vi "Move new unbundler WRT Terminal.vi"(6 "Offset":i32=-15, 8 "error in":errorcluster, 9 "New objects created":refnum<vi>[](array[refnum]), 10 "Named Un/Bundler Ref":refnum<vi>, 11 "Terminal Data Cluster":T1) -> (0 "error out":errorcluster)   [LabVIEW 2023]
doc: "Because a bundler will expand to the right once its labels are set, and we want to place the bundler to the left of a sink terminal, this VI will adjust the new objects created (a bundler and optional constant) to be positioned the correct offset from the affected terminal. Offset is by default -15px.\n\nThis is not needed for bundlers on source terminals, so we ignore those."
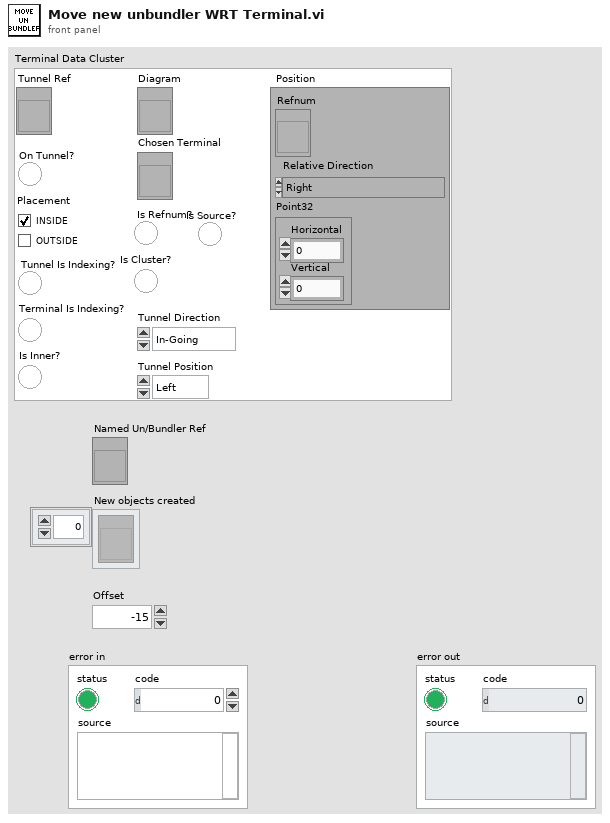
[diagram p1: front panel]
types:
  T1 = cluster{"Tunnel Ref":refnum<vi>, "On Tunnel?":bool, "Placement":enum32{"Choice 1", "Choice 2"}, "Tunnel Is Indexing?":bool, "Diagram":refnum<vi>, "Position":cluster{"Refnum":refnum<vi>, "Relative Direction":enum32{"Right", "Left", "Top", "Bottom", "Top Right", "Top Left", "Bottom Right", "Bottom Left"}, "Point32":cluster{"Horizontal":i32, "Vertical":i32}}, "Chosen Terminal":refnum<vi>, "Is Refnum?":bool, "Is Cluster?":bool, "Is Source?":bool, "Tunnel Direction":enum16{"In-Going", "Out-Going"}, "Tunnel Position":enum16{"Left", "Top", "Right", "Bottom"}, "Is Inner?":bool, "Terminal Is Indexing?":bool}
  T2 = typedef "LVPositionTypeDef.ctl" = cluster{"Left":i32, "Top":i32}
  T3 = typedef "LVRectTypeDef.ctl" = cluster{"Left":i16, "Top":i16, "Right":i16, "Bottom":i16}
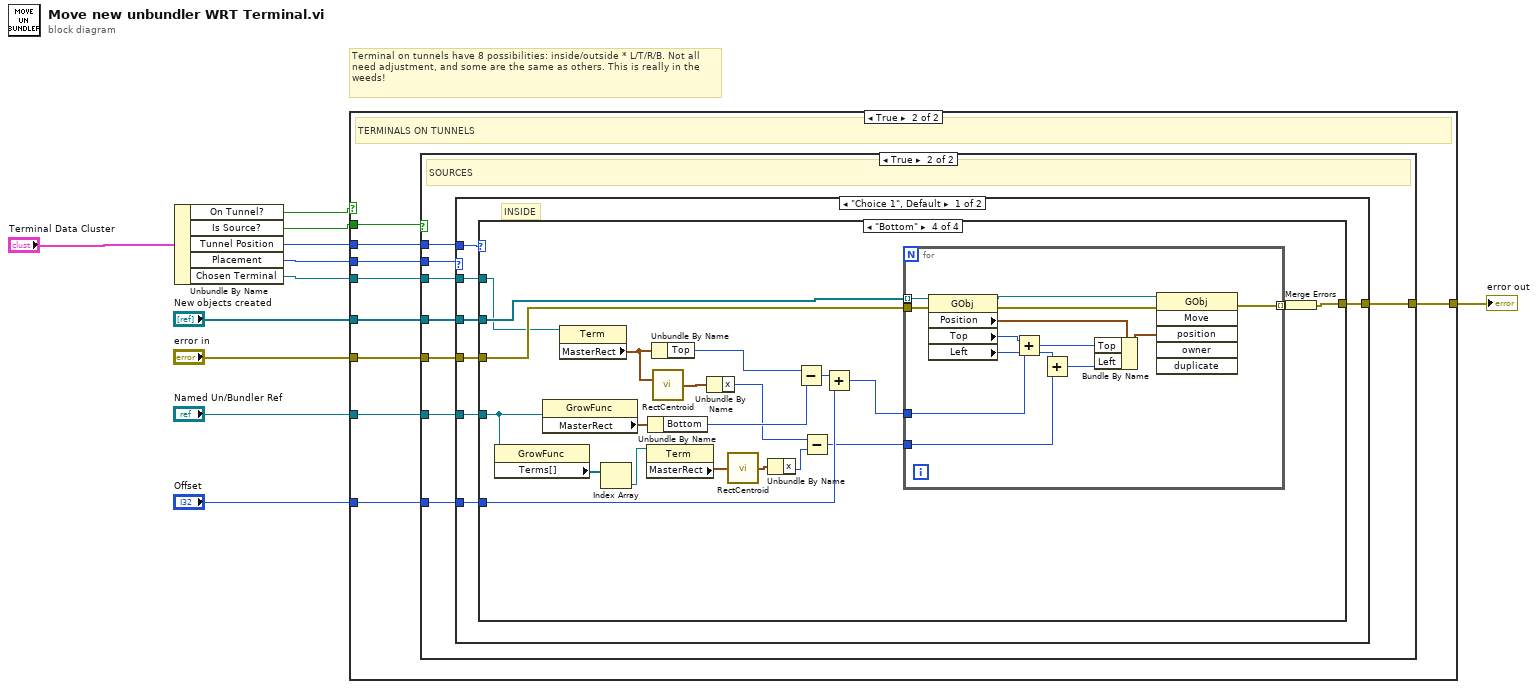
[diagram p0: block diagram]
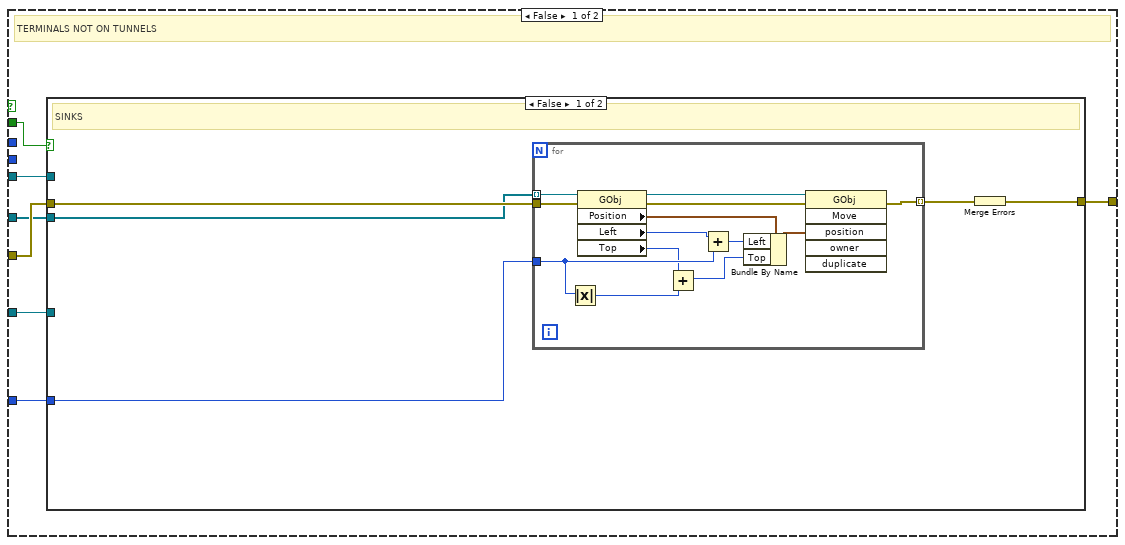
[diagram p2: hidden frame]
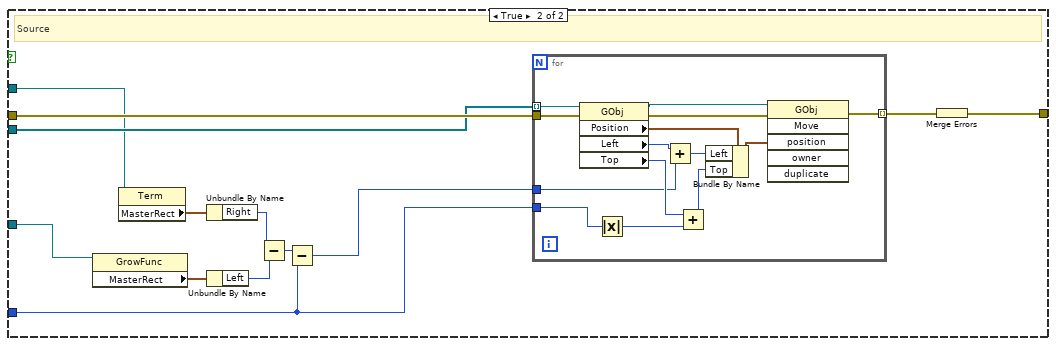
[diagram p3: hidden frame]
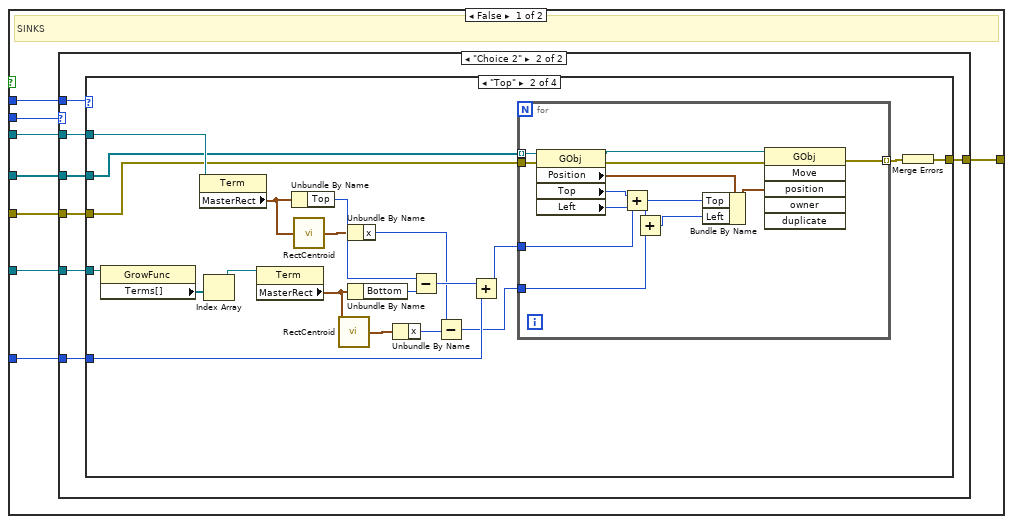
[diagram p4: hidden frame]
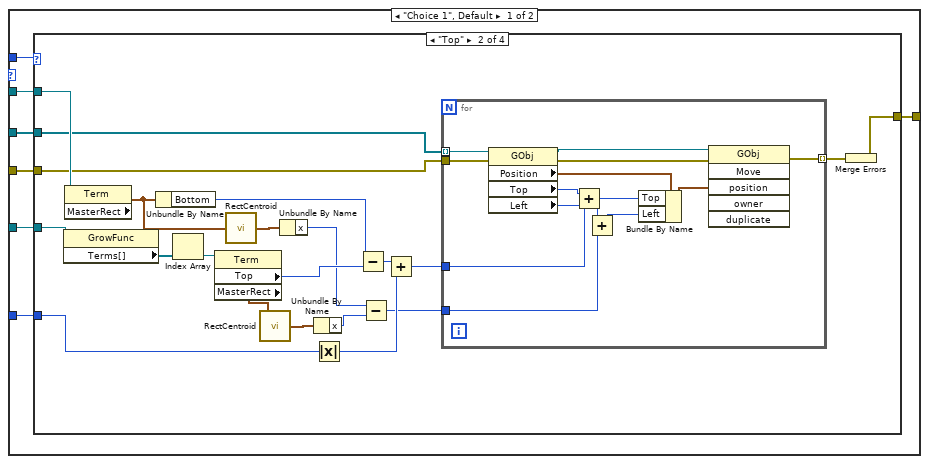
[diagram p5: hidden frame]
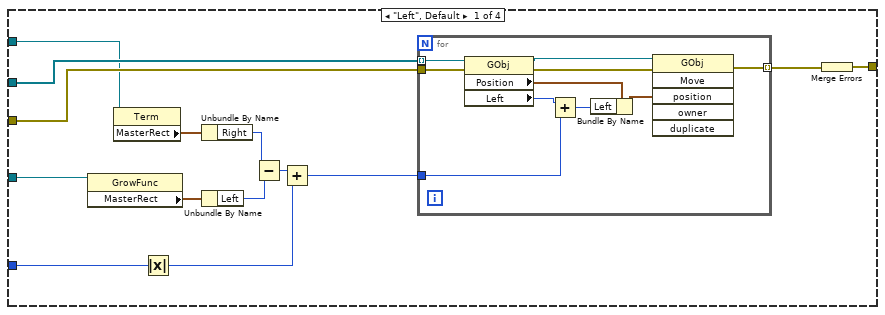
[diagram p6: hidden frame]
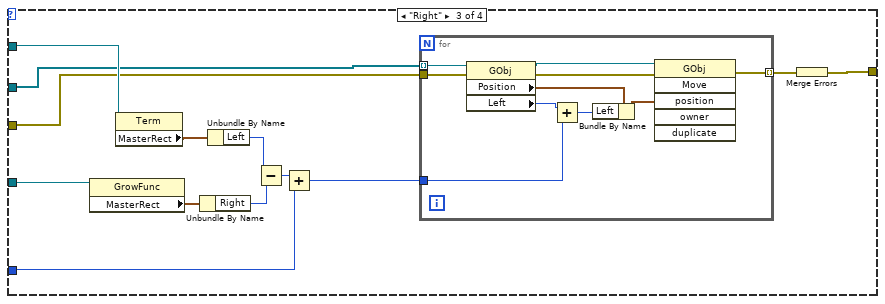
[diagram p7: hidden frame]
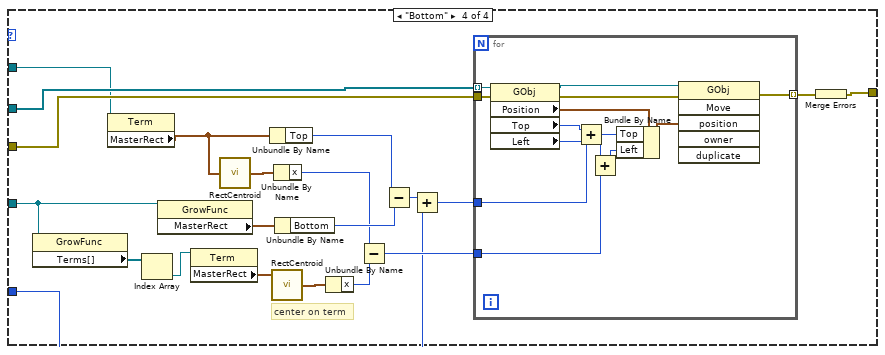
[diagram p8: hidden frame]
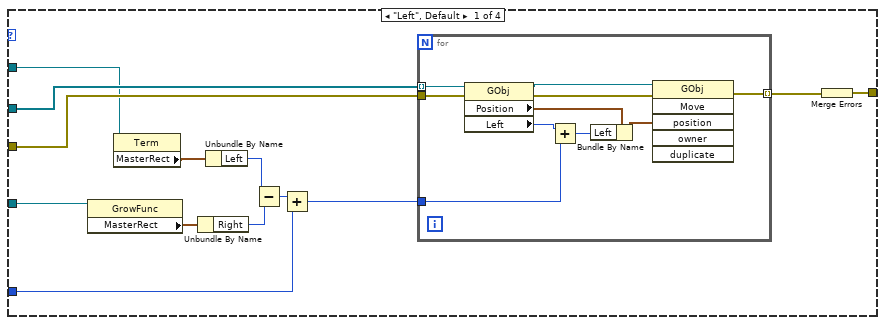
[diagram p9: hidden frame]
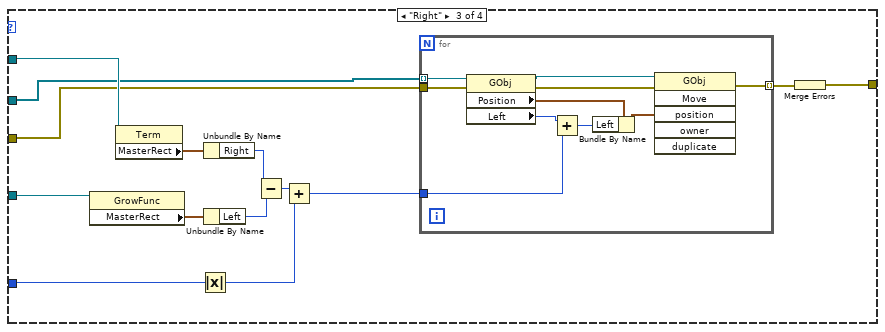
[diagram p10: hidden frame]
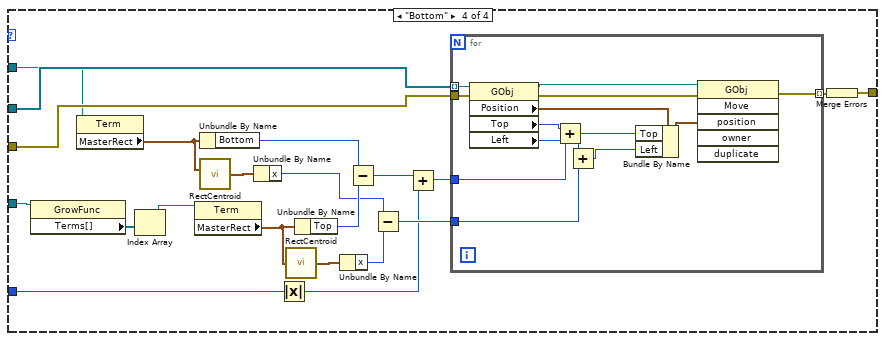
[diagram p11: hidden frame]
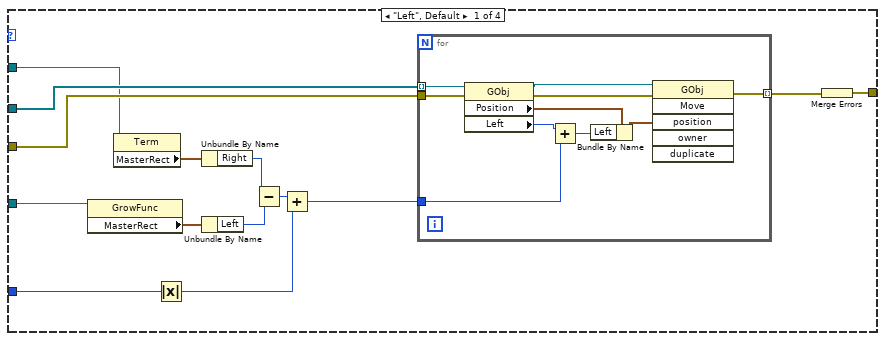
[diagram p12: hidden frame]
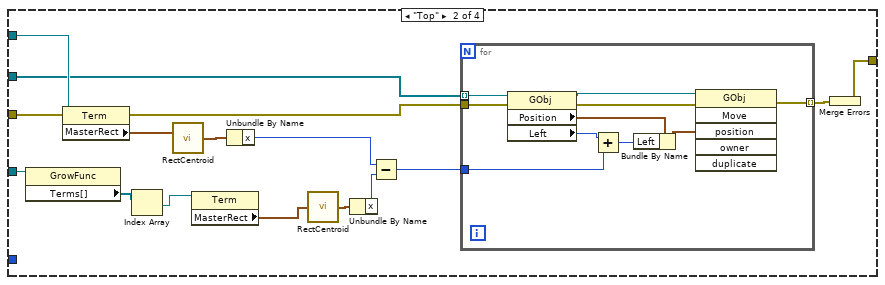
[diagram p13: hidden frame]
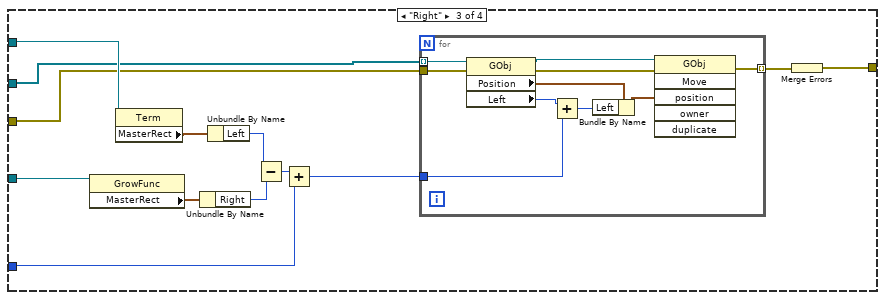
[diagram p14: hidden frame]
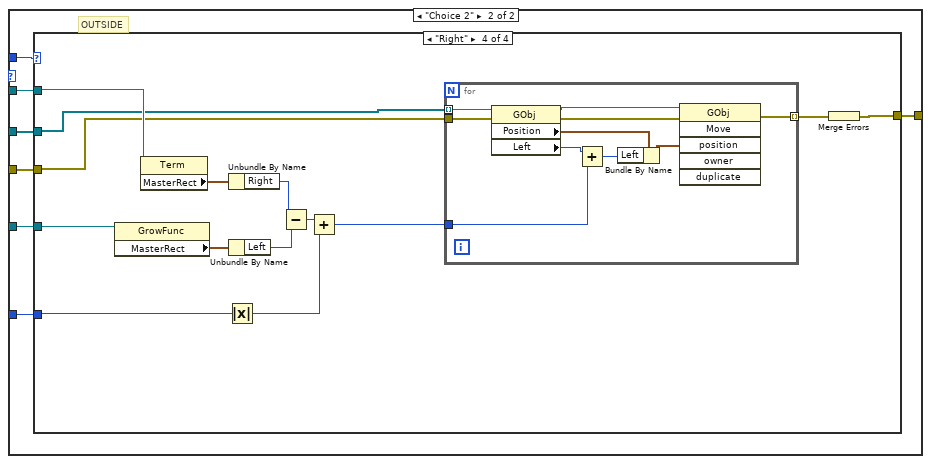
[diagram p15: hidden frame]
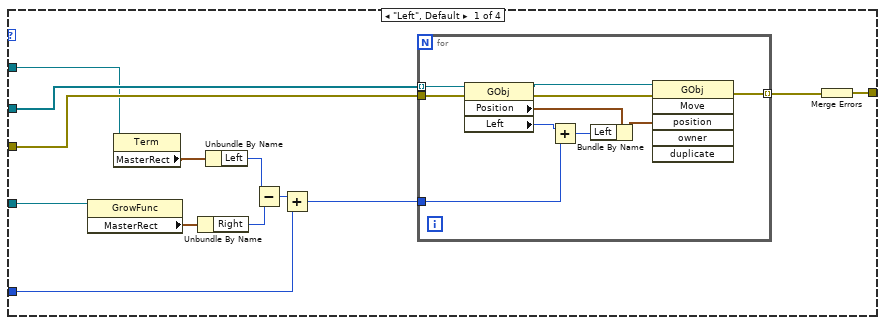
[diagram p16: hidden frame]
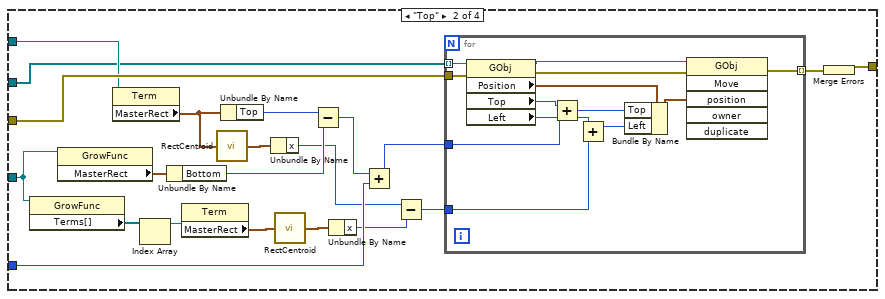
[diagram p17: hidden frame]
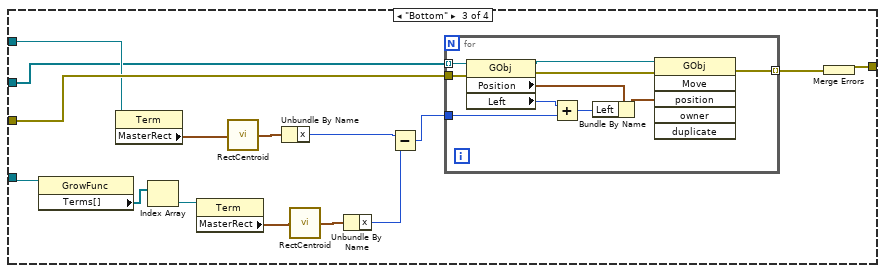
[diagram p18: hidden frame]
diagram:
  # "Terminal on tunnels have 8 possibilities: inside/outside * L/T/R/B. Not all need adjustment, and some are the same as others. This is really in the weeds!"
  n1 = Unbundle By Name("Terminal Data Cluster") -> ("On Tunnel?"=w5:bool, "Is Source?"=w4:bool, "Tunnel Position"=w3:enum16{"Left", "Top", "Right", "Bottom"}, "Placement"=w2:enum32{"Choice 1", "Choice 2"}, "Chosen Terminal"=w6:refnum<vi>)
  n2 = case shown="True" w5 {
    tunnel: "Offset" -> [w18 w64]
    tunnel: "Named Un/Bundler Ref" -> [w17 w66]
    tunnel: [w16 w69] -> w9
    tunnel: "error in" -> [w15 w68]
    tunnel: w4 -> [w14 w72]
    tunnel: w6 -> [w13 w65]
    tunnel: w3 -> [_ w71]
    tunnel: w2 -> [_ w70]
    tunnel: "New objects created" -> [w12 w67]
    frame False {
      # "TERMINALS NOT ON TUNNELS"
      n3 = case shown="False" w14 {
        tunnel: w18 -> [w23 w38]
        tunnel: w17 -> [_ w39]
        tunnel: w13 -> [_ w40]
        tunnel: [w21 w48] -> w16
        tunnel: w15 -> [w20 w47]
        tunnel: w12 -> [w19 w46]
        frame False {
          # "SINKS"
          n4 = for {
            tunnel: w19 -> [w36] mode=indexing
            tunnel: w23 -> [w27]
            tunnel: w20 -> [w30]
            tunnel: [w28] -> w22 mode=indexing
            n5 = Absolute Value(x=w27) -> (abs(x)=w24:i32)
            n6 = property class="GObj"(reference=w36, error in=w30) -> (reference out=w35:refnum<vi>, error out=w29:errorcluster, "Position"=w33:T2, "Left"=w34:i32, "Top"=w26:i32)
            n7 = Add(x=w26, y=w24) -> (x+y=w25:i32)
            n8 = Add(x=w34, y=w27) -> (x+y=w32:i32)
            n9 = Bundle By Name(cluster=w33, "Left"=w32, "Top"=w25) -> (w31:T2)
            n10 = invoke class="GObj" method="Move"(reference=w35, error in=w29, "position"=w31) -> (error out=w28:errorcluster)  [unwired: 3 in, 5 out]
          }
          n11 = Merge Errors(w22) -> (w21:errorcluster)
        }
        frame True {
          # "Source"
          n12 = property class="GrowFunc"(reference=w39) -> ("MasterRect"=w44:T3)  [unwired: 1 in, 2 out]
          n13 = property class="Term"(reference=w40) -> ("MasterRect"=w43:T3)  [unwired: 1 in, 2 out]
          n14 = Unbundle By Name(w43) -> ("Right"=w42:i16)
          n15 = Unbundle By Name(w44) -> ("Left"=w41:i16)
          n16 = Subtract(x=w42, y=w41) -> (x-y=w45:i16)
          n17 = Subtract(x=w45, y=w38) -> (x-y=w37:i32)
          n18 = for {
            tunnel: w46 -> [w63] mode=indexing
            tunnel: w38 -> [w50]
            tunnel: w47 -> [w57]
            tunnel: [w55] -> w49 mode=indexing
            tunnel: w37 -> [w51]
            n19 = property class="GObj"(reference=w63, error in=w57) -> (reference out=w62:refnum<vi>, error out=w56:errorcluster, "Position"=w60:T2, "Left"=w61:i32, "Top"=w53:i32)
            n20 = Absolute Value(x=w50) -> (abs(x)=w54:i32)
            n21 = Add(x=w61, y=w51) -> (x+y=w59:i32)
            n22 = Add(x=w53, y=w54) -> (x+y=w52:i32)
            n23 = Bundle By Name(cluster=w60, "Left"=w59, "Top"=w52) -> (w58:T2)
            n24 = invoke class="GObj" method="Move"(reference=w62, error in=w56, "position"=w58) -> (error out=w55:errorcluster)  [unwired: 3 in, 5 out]
          }
          n25 = Merge Errors(w49) -> (w48:errorcluster)
        }
      }
    }
    frame True {
      # "TERMINALS ON TUNNELS"
      n26 = case shown="True" w72 {
        tunnel: w71 -> [w80 w331]
        tunnel: w70 -> [w79 w330]
        tunnel: [w78 w324] -> w69
        tunnel: w68 -> [w77 w327]
        tunnel: w67 -> [w76 w328]
        tunnel: w66 -> [w75 w326]
        tunnel: w65 -> [w74 w329]
        tunnel: w64 -> [w73 w325]
        frame False {
          # "SINKS"
          n27 = case shown="\"Choice 2\"" w79 {
            tunnel: w80 -> [w87 w209]
            tunnel: [w81 w208] -> w78
            tunnel: w77 -> [w84 w207]
            tunnel: w76 -> [w85 w206]
            tunnel: w75 -> [w82 w205]
            tunnel: w74 -> [w86 w204]
            tunnel: w73 -> [w83 w203]
            frame "Choice 1", Default {
              n28 = case shown="\"Top\"" w87 {
                tunnel: [w96 w126 w158 w180] -> w81
                tunnel: w84 -> [w100 w128 w155 w182]
                tunnel: w85 -> [w101 w127 w156 w183]
                tunnel: w82 -> [w99 w125 w154 w179]
                tunnel: w86 -> [w98 w129 w157 w181]
                tunnel: w83 -> [w97 w120 w153 w173]
                frame "Left", Default {
                  n29 = property class="GrowFunc"(reference=w99) -> ("MasterRect"=w94:T3)  [unwired: 1 in, 2 out]
                  n30 = property class="Term"(reference=w98) -> ("MasterRect"=w93:T3)  [unwired: 1 in, 2 out]
                  n31 = Absolute Value(x=w97) -> (abs(x)=w88:i32)
                  n32 = Unbundle By Name(w93) -> ("Right"=w92:i16)
                  n33 = Unbundle By Name(w94) -> ("Left"=w91:i16)
                  n34 = Subtract(x=w92, y=w91) -> (x-y=w95:i16)
                  n35 = Add(x=w95, y=w88) -> (x+y=w90:i32)
                  n36 = for {
                    tunnel: w90 -> [w109]
                    tunnel: [w104] -> w89 mode=indexing
                    tunnel: w101 -> [w103] mode=indexing
                    tunnel: w100 -> [w102]
                    n37 = property class="GObj"(reference=w103, error in=w102) -> (reference out=w111:refnum<vi>, error out=w105:errorcluster, "Position"=w108:T2, "Left"=w110:i32)
                    n38 = Add(x=w110, y=w109) -> (x+y=w107:i32)
                    n39 = Bundle By Name(cluster=w108, "Left"=w107) -> (w106:T2)
                    n40 = invoke class="GObj" method="Move"(reference=w111, error in=w105, "position"=w106) -> (error out=w104:errorcluster)  [unwired: 3 in, 5 out]
                  }
                  n41 = Merge Errors(w89) -> (w96:errorcluster)
                }
                frame "Top" {
                  n42 = property class="GrowFunc"(reference=w125) -> ("Terms[]"=w124:refnum<vi>[])  [unwired: 1 in, 2 out]
                  n43 = property class="Term"(reference=w129) -> ("MasterRect"=w114:T3)  [unwired: 1 in, 2 out]
                  n44 = Unbundle By Name(w114) -> ("Bottom"=w118:i16)
                  n45 = Index Array(array=w124) -> (element=w123:refnum<vi>)  [unwired: 1 in]
                  n46 = property class="Term"(reference=w123) -> ("Top"=w122:i32, "MasterRect"=w115:T3)  [unwired: 1 in, 2 out]
                  n47 = call <vilib>:"RectCentroid.vi"("rect"=w114) -> ("point"=w117:cluster{"x":i16, "y":i16})
                  n48 = call <vilib>:"RectCentroid.vi"("rect"=w115) -> ("point"=w116:cluster{"x":i16, "y":i16})
                  n49 = Unbundle By Name(w117) -> ("x"=w113:i16)
                  n50 = Unbundle By Name(w116) -> ("x"=w112:i16)
                  n51 = Absolute Value(x=w120) -> (abs(x)=w121:i32)
                  n52 = Subtract(x=w118, y=w122) -> (x-y=w132:i32)
                  n53 = Subtract(x=w113, y=w112) -> (x-y=w119:i16)
                  n54 = Add(x=w132, y=w121) -> (x+y=w131:i32)
                  n55 = for {
                    tunnel: w131 -> [w143]
                    tunnel: [w138] -> w130 mode=indexing
                    tunnel: w128 -> [w137]
                    tunnel: w127 -> [w136] mode=indexing
                    tunnel: w119 -> [w134]
                    n56 = property class="GObj"(reference=w136, error in=w137) -> (reference out=w145:refnum<vi>, error out=w139:errorcluster, "Position"=w142:T2, "Top"=w144:i32, "Left"=w135:i32)
                    n57 = Add(x=w144, y=w143) -> (x+y=w141:i32)
                    n58 = Add(x=w135, y=w134) -> (x+y=w133:i32)
                    n59 = Bundle By Name(cluster=w142, "Top"=w141, "Left"=w133) -> (w140:T2)
                    n60 = invoke class="GObj" method="Move"(reference=w145, error in=w139, "position"=w140) -> (error out=w138:errorcluster)  [unwired: 3 in, 5 out]
                  }
                  n61 = Merge Errors(w130) -> (w126:errorcluster)
                }
                frame "Right" {
                  n62 = property class="GrowFunc"(reference=w154) -> ("MasterRect"=w151:T3)  [unwired: 1 in, 2 out]
                  n63 = property class="Term"(reference=w157) -> ("MasterRect"=w150:T3)  [unwired: 1 in, 2 out]
                  n64 = Unbundle By Name(w151) -> ("Right"=w148:i16)
                  n65 = Unbundle By Name(w150) -> ("Left"=w149:i16)
                  n66 = Subtract(x=w149, y=w148) -> (x-y=w152:i16)
                  n67 = Add(x=w152, y=w153) -> (x+y=w147:i32)
                  n68 = for {
                    tunnel: w156 -> [w168] mode=indexing
                    tunnel: w147 -> [w165]
                    tunnel: w155 -> [w161]
                    tunnel: [w159] -> w146 mode=indexing
                    n69 = property class="GObj"(reference=w168, error in=w161) -> (reference out=w167:refnum<vi>, error out=w160:errorcluster, "Position"=w164:T2, "Left"=w166:i32)
                    n70 = Add(x=w166, y=w165) -> (x+y=w163:i32)
                    n71 = Bundle By Name(cluster=w164, "Left"=w163) -> (w162:T2)
                    n72 = invoke class="GObj" method="Move"(reference=w167, error in=w160, "position"=w162) -> (error out=w159:errorcluster)  [unwired: 3 in, 5 out]
                  }
                  n73 = Merge Errors(w146) -> (w158:errorcluster)
                }
                frame "Bottom" {
                  # "center on term"
                  n74 = property class="GrowFunc"(reference=w179) -> ("Terms[]"=w178:refnum<vi>[])  [unwired: 1 in, 2 out]
                  n75 = property class="Term"(reference=w181) -> ("MasterRect"=w174:T3)  [unwired: 1 in, 2 out]
                  n76 = Index Array(array=w178) -> (element=w177:refnum<vi>)  [unwired: 1 in]
                  n77 = property class="GrowFunc"(reference=w179) -> ("MasterRect"=w188:T3)  [unwired: 1 in, 2 out]
                  n78 = property class="Term"(reference=w177) -> ("MasterRect"=w172:T3)  [unwired: 1 in, 2 out]
                  n79 = call <vilib>:"RectCentroid.vi"("rect"=w174) -> ("point"=w175:cluster{"x":i16, "y":i16})
                  n80 = Unbundle By Name(w174) -> ("Top"=w187:i16)
                  n81 = call <vilib>:"RectCentroid.vi"("rect"=w172) -> ("point"=w171:cluster{"x":i16, "y":i16})
                  n82 = Unbundle By Name(w175) -> ("x"=w170:i16)
                  n83 = Unbundle By Name(w188) -> ("Bottom"=w186:i16)
                  n84 = Unbundle By Name(w171) -> ("x"=w169:i16)
                  n85 = Subtract(x=w170, y=w169) -> (x-y=w176:i16)
                  n86 = Subtract(x=w187, y=w186) -> (x-y=w189:i16)
                  n87 = Add(x=w189, y=w173) -> (x+y=w185:i32)
                  n88 = for {
                    tunnel: w183 -> [w202] mode=indexing
                    tunnel: w185 -> [w199]
                    tunnel: w182 -> [w195]
                    tunnel: [w193] -> w184 mode=indexing
                    tunnel: w176 -> [w191]
                    n89 = property class="GObj"(reference=w202, error in=w195) -> (reference out=w201:refnum<vi>, error out=w194:errorcluster, "Position"=w198:T2, "Top"=w200:i32, "Left"=w192:i32)
                    n90 = Add(x=w200, y=w199) -> (x+y=w197:i32)
                    n91 = Add(x=w192, y=w191) -> (x+y=w190:i32)
                    n92 = Bundle By Name(cluster=w198, "Top"=w197, "Left"=w190) -> (w196:T2)
                    n93 = invoke class="GObj" method="Move"(reference=w201, error in=w194, "position"=w196) -> (error out=w193:errorcluster)  [unwired: 3 in, 5 out]
                  }
                  n94 = Merge Errors(w184) -> (w180:errorcluster)
                }
              }
            }
            frame "Choice 2" {
              n95 = case shown="\"Top\"" w209 {
                tunnel: [w210 w244 w279 w304] -> w208
                tunnel: w207 -> [w214 w246 w276 w303]
                tunnel: w206 -> [w215 w245 w277 w302]
                tunnel: w205 -> [w213 w242 w275 w300]
                tunnel: w204 -> [w212 w247 w278 w301]
                tunnel: w203 -> [w211 w243 w274 w299]
                frame "Left", Default {
                  n96 = property class="GrowFunc"(reference=w213) -> ("MasterRect"=w221:T3)  [unwired: 1 in, 2 out]
                  n97 = property class="Term"(reference=w212) -> ("MasterRect"=w220:T3)  [unwired: 1 in, 2 out]
                  n98 = Unbundle By Name(w221) -> ("Right"=w218:i16)
                  n99 = Unbundle By Name(w220) -> ("Left"=w219:i16)
                  n100 = Subtract(x=w219, y=w218) -> (x-y=w222:i16)
                  n101 = Add(x=w222, y=w211) -> (x+y=w217:i32)
                  n102 = for {
                    tunnel: w217 -> [w230]
                    tunnel: [w225] -> w216 mode=indexing
                    tunnel: w215 -> [w224] mode=indexing
                    tunnel: w214 -> [w223]
                    n103 = property class="GObj"(reference=w224, error in=w223) -> (reference out=w232:refnum<vi>, error out=w226:errorcluster, "Position"=w229:T2, "Left"=w231:i32)
                    n104 = Add(x=w231, y=w230) -> (x+y=w228:i32)
                    n105 = Bundle By Name(cluster=w229, "Left"=w228) -> (w227:T2)
                    n106 = invoke class="GObj" method="Move"(reference=w232, error in=w226, "position"=w227) -> (error out=w225:errorcluster)  [unwired: 3 in, 5 out]
                  }
                  n107 = Merge Errors(w216) -> (w210:errorcluster)
                }
                frame "Top" {
                  n108 = property class="GrowFunc"(reference=w242) -> ("Terms[]"=w234:refnum<vi>[])  [unwired: 1 in, 2 out]
                  n109 = property class="Term"(reference=w247) -> ("MasterRect"=w239:T3)  [unwired: 1 in, 2 out]
                  n110 = Index Array(array=w234) -> (element=w233:refnum<vi>)  [unwired: 1 in]
                  n111 = property class="Term"(reference=w233) -> ("MasterRect"=w236:T3)  [unwired: 1 in, 2 out]
                  n112 = Unbundle By Name(w239) -> ("Top"=w251:i16)
                  n113 = call <vilib>:"RectCentroid.vi"("rect"=w239) -> ("point"=w240:cluster{"x":i16, "y":i16})
                  n114 = call <vilib>:"RectCentroid.vi"("rect"=w236) -> ("point"=w237:cluster{"x":i16, "y":i16})
                  n115 = Unbundle By Name(w240) -> ("x"=w238:i16)
                  n116 = Unbundle By Name(w236) -> ("Bottom"=w250:i16)
                  n117 = Unbundle By Name(w237) -> ("x"=w235:i16)
                  n118 = Subtract(x=w251, y=w250) -> (x-y=w252:i16)
                  n119 = Subtract(x=w238, y=w235) -> (x-y=w241:i16)
                  n120 = Add(x=w252, y=w243) -> (x+y=w249:i32)
                  n121 = for {
                    tunnel: w249 -> [w263]
                    tunnel: [w258] -> w248 mode=indexing
                    tunnel: w246 -> [w257]
                    tunnel: w245 -> [w256] mode=indexing
                    tunnel: w241 -> [w254]
                    n122 = property class="GObj"(reference=w256, error in=w257) -> (reference out=w265:refnum<vi>, error out=w259:errorcluster, "Position"=w262:T2, "Top"=w264:i32, "Left"=w255:i32)
                    n123 = Add(x=w264, y=w263) -> (x+y=w261:i32)
                    n124 = Add(x=w255, y=w254) -> (x+y=w253:i32)
                    n125 = Bundle By Name(cluster=w262, "Top"=w261, "Left"=w253) -> (w260:T2)
                    n126 = invoke class="GObj" method="Move"(reference=w265, error in=w259, "position"=w260) -> (error out=w258:errorcluster)  [unwired: 3 in, 5 out]
                  }
                  n127 = Merge Errors(w248) -> (w244:errorcluster)
                }
                frame "Right" {
                  n128 = property class="GrowFunc"(reference=w275) -> ("MasterRect"=w272:T3)  [unwired: 1 in, 2 out]
                  n129 = property class="Term"(reference=w278) -> ("MasterRect"=w271:T3)  [unwired: 1 in, 2 out]
                  n130 = Absolute Value(x=w274) -> (abs(x)=w266:i32)
                  n131 = Unbundle By Name(w271) -> ("Right"=w270:i16)
                  n132 = Unbundle By Name(w272) -> ("Left"=w269:i16)
                  n133 = Subtract(x=w270, y=w269) -> (x-y=w273:i16)
                  n134 = Add(x=w273, y=w266) -> (x+y=w268:i32)
                  n135 = for {
                    tunnel: w277 -> [w289] mode=indexing
                    tunnel: w268 -> [w286]
                    tunnel: w276 -> [w282]
                    tunnel: [w280] -> w267 mode=indexing
                    n136 = property class="GObj"(reference=w289, error in=w282) -> (reference out=w288:refnum<vi>, error out=w281:errorcluster, "Position"=w285:T2, "Left"=w287:i32)
                    n137 = Add(x=w287, y=w286) -> (x+y=w284:i32)
                    n138 = Bundle By Name(cluster=w285, "Left"=w284) -> (w283:T2)
                    n139 = invoke class="GObj" method="Move"(reference=w288, error in=w281, "position"=w283) -> (error out=w280:errorcluster)  [unwired: 3 in, 5 out]
                  }
                  n140 = Merge Errors(w267) -> (w279:errorcluster)
                }
                frame "Bottom" {
                  n141 = property class="GrowFunc"(reference=w300) -> ("Terms[]"=w291:refnum<vi>[])  [unwired: 1 in, 2 out]
                  n142 = property class="Term"(reference=w301) -> ("MasterRect"=w293:T3)  [unwired: 1 in, 2 out]
                  n143 = Index Array(array=w291) -> (element=w290:refnum<vi>)  [unwired: 1 in]
                  n144 = property class="Term"(reference=w290) -> ("MasterRect"=w296:T3)  [unwired: 1 in, 2 out]
                  n145 = Unbundle By Name(w293) -> ("Bottom"=w309:i16)
                  n146 = call <vilib>:"RectCentroid.vi"("rect"=w293) -> ("point"=w294:cluster{"x":i16, "y":i16})
                  n147 = Unbundle By Name(w294) -> ("x"=w292:i16)
                  n148 = Absolute Value(x=w299) -> (abs(x)=w298:i32)
                  n149 = call <vilib>:"RectCentroid.vi"("rect"=w296) -> ("point"=w297:cluster{"x":i16, "y":i16})
                  n150 = Unbundle By Name(w296) -> ("Top"=w308:i16)
                  n151 = Unbundle By Name(w297) -> ("x"=w295:i16)
                  n152 = Subtract(x=w309, y=w308) -> (x-y=w310:i16)
                  n153 = Subtract(x=w292, y=w295) -> (x-y=w305:i16)
                  n154 = Add(x=w310, y=w298) -> (x+y=w307:i32)
                  n155 = for {
                    tunnel: w307 -> [w321]
                    tunnel: [w316] -> w306 mode=indexing
                    tunnel: w303 -> [w315]
                    tunnel: w302 -> [w314] mode=indexing
                    tunnel: w305 -> [w312]
                    n156 = property class="GObj"(reference=w314, error in=w315) -> (reference out=w323:refnum<vi>, error out=w317:errorcluster, "Position"=w320:T2, "Top"=w322:i32, "Left"=w313:i32)
                    n157 = Add(x=w322, y=w321) -> (x+y=w319:i32)
                    n158 = Add(x=w313, y=w312) -> (x+y=w311:i32)
                    n159 = Bundle By Name(cluster=w320, "Top"=w319, "Left"=w311) -> (w318:T2)
                    n160 = invoke class="GObj" method="Move"(reference=w323, error in=w317, "position"=w318) -> (error out=w316:errorcluster)  [unwired: 3 in, 5 out]
                  }
                  n161 = Merge Errors(w306) -> (w304:errorcluster)
                }
              }
            }
          }
        }
        frame True {
          # "SOURCES"
          n162 = case shown="\"Choice 1\", Default" w330 {
            tunnel: w331 -> [w338 w451]
            tunnel: w329 -> [w337 w450]
            tunnel: w328 -> [w336 w449]
            tunnel: w327 -> [w335 w448]
            tunnel: w326 -> [w334 w447]
            tunnel: w325 -> [w333 w446]
            tunnel: [w332 w445] -> w324
            frame "Choice 1", Default {
              # "INSIDE"
              n163 = case shown="\"Bottom\"" w338 {
                tunnel: [w347 w374 w400 w422] -> w332
                tunnel: w335 -> [w351 w376 w397 w425]
                tunnel: w336 -> [w352 w375 w398 w426]
                tunnel: w334 -> [w350 w365 w396 w413]
                tunnel: w337 -> [w349 w377 w399 w424]
                tunnel: w333 -> [w348 _ w395 w423]
                frame "Left", Default {
                  n164 = property class="GrowFunc"(reference=w350) -> ("MasterRect"=w345:T3)  [unwired: 1 in, 2 out]
                  n165 = property class="Term"(reference=w349) -> ("MasterRect"=w344:T3)  [unwired: 1 in, 2 out]
                  n166 = Absolute Value(x=w348) -> (abs(x)=w340:i32)
                  n167 = Unbundle By Name(w344) -> ("Right"=w343:i16)
                  n168 = Unbundle By Name(w345) -> ("Left"=w342:i16)
                  n169 = Subtract(x=w343, y=w342) -> (x-y=w346:i16)
                  n170 = Add(x=w346, y=w340) -> (x+y=w339:i32)
                  n171 = for {
                    tunnel: w339 -> [w360]
                    tunnel: [w355] -> w341 mode=indexing
                    tunnel: w352 -> [w354] mode=indexing
                    tunnel: w351 -> [w353]
                    n172 = property class="GObj"(reference=w354, error in=w353) -> (reference out=w362:refnum<vi>, error out=w356:errorcluster, "Position"=w359:T2, "Left"=w361:i32)
                    n173 = Add(x=w361, y=w360) -> (x+y=w358:i32)
                    n174 = Bundle By Name(cluster=w359, "Left"=w358) -> (w357:T2)
                    n175 = invoke class="GObj" method="Move"(reference=w362, error in=w356, "position"=w357) -> (error out=w355:errorcluster)  [unwired: 3 in, 5 out]
                  }
                  n176 = Merge Errors(w341) -> (w347:errorcluster)
                }
                frame "Top" {
                  n177 = property class="GrowFunc"(reference=w365) -> ("Terms[]"=w364:refnum<vi>[])  [unwired: 1 in, 2 out]
                  n178 = property class="Term"(reference=w377) -> ("MasterRect"=w371:T3)  [unwired: 1 in, 2 out]
                  n179 = Index Array(array=w364) -> (element=w363:refnum<vi>)  [unwired: 1 in]
                  n180 = call <vilib>:"RectCentroid.vi"("rect"=w371) -> ("point"=w372:cluster{"x":i16, "y":i16})
                  n181 = property class="Term"(reference=w363) -> ("MasterRect"=w369:T3)  [unwired: 1 in, 2 out]
                  n182 = Unbundle By Name(w372) -> ("x"=w370:i16)
                  n183 = call <vilib>:"RectCentroid.vi"("rect"=w369) -> ("point"=w368:cluster{"x":i16, "y":i16})
                  n184 = Unbundle By Name(w368) -> ("x"=w367:i16)
                  n185 = Subtract(x=w370, y=w367) -> (x-y=w366:i16)
                  n186 = for {
                    tunnel: [w381] -> w373 mode=indexing
                    tunnel: w376 -> [w380]
                    tunnel: w375 -> [w379] mode=indexing
                    tunnel: w366 -> [w378]
                    n187 = property class="GObj"(reference=w379, error in=w380) -> (reference out=w387:refnum<vi>, error out=w382:errorcluster, "Position"=w385:T2, "Left"=w386:i32)
                    n188 = Add(x=w386, y=w378) -> (x+y=w384:i32)
                    n189 = Bundle By Name(cluster=w385, "Left"=w384) -> (w383:T2)
                    n190 = invoke class="GObj" method="Move"(reference=w387, error in=w382, "position"=w383) -> (error out=w381:errorcluster)  [unwired: 3 in, 5 out]
                  }
                  n191 = Merge Errors(w373) -> (w374:errorcluster)
                }
                frame "Right" {
                  n192 = property class="GrowFunc"(reference=w396) -> ("MasterRect"=w393:T3)  [unwired: 1 in, 2 out]
                  n193 = property class="Term"(reference=w399) -> ("MasterRect"=w392:T3)  [unwired: 1 in, 2 out]
                  n194 = Unbundle By Name(w393) -> ("Right"=w390:i16)
                  n195 = Unbundle By Name(w392) -> ("Left"=w391:i16)
                  n196 = Subtract(x=w391, y=w390) -> (x-y=w394:i16)
                  n197 = Add(x=w394, y=w395) -> (x+y=w388:i32)
                  n198 = for {
                    tunnel: w398 -> [w410] mode=indexing
                    tunnel: w388 -> [w407]
                    tunnel: w397 -> [w403]
                    tunnel: [w401] -> w389 mode=indexing
                    n199 = property class="GObj"(reference=w410, error in=w403) -> (reference out=w409:refnum<vi>, error out=w402:errorcluster, "Position"=w406:T2, "Left"=w408:i32)
                    n200 = Add(x=w408, y=w407) -> (x+y=w405:i32)
                    n201 = Bundle By Name(cluster=w406, "Left"=w405) -> (w404:T2)
                    n202 = invoke class="GObj" method="Move"(reference=w409, error in=w402, "position"=w404) -> (error out=w401:errorcluster)  [unwired: 3 in, 5 out]
                  }
                  n203 = Merge Errors(w389) -> (w400:errorcluster)
                }
                frame "Bottom" {
                  n204 = property class="GrowFunc"(reference=w413) -> ("Terms[]"=w414:refnum<vi>[])  [unwired: 1 in, 2 out]
                  n205 = property class="GrowFunc"(reference=w413) -> ("MasterRect"=w419:T3)  [unwired: 1 in, 2 out]
                  n206 = property class="Term"(reference=w424) -> ("MasterRect"=w417:T3)  [unwired: 1 in, 2 out]
                  n207 = Index Array(array=w414) -> (element=w412:refnum<vi>)  [unwired: 1 in]
                  n208 = property class="Term"(reference=w412) -> ("MasterRect"=w411:T3)  [unwired: 1 in, 2 out]
                  n209 = Unbundle By Name(w419) -> ("Bottom"=w429:i16)
                  n210 = Unbundle By Name(w417) -> ("Top"=w430:i16)
                  n211 = call <vilib>:"RectCentroid.vi"("rect"=w417) -> ("point"=w418:cluster{"x":i16, "y":i16})
                  n212 = Unbundle By Name(w418) -> ("x"=w416:i16)
                  n213 = call <vilib>:"RectCentroid.vi"("rect"=w411) -> ("point"=w420:cluster{"x":i16, "y":i16})
                  n214 = Unbundle By Name(w420) -> ("x"=w415:i16)
                  n215 = Subtract(x=w430, y=w429) -> (x-y=w431:i16)
                  n216 = Subtract(x=w416, y=w415) -> (x-y=w421:i16)
                  n217 = Add(x=w431, y=w423) -> (x+y=w428:i32)
                  n218 = for {
                    tunnel: w426 -> [w444] mode=indexing
                    tunnel: w428 -> [w441]
                    tunnel: w425 -> [w437]
                    tunnel: [w435] -> w427 mode=indexing
                    tunnel: w421 -> [w432]
                    n219 = property class="GObj"(reference=w444, error in=w437) -> (reference out=w443:refnum<vi>, error out=w436:errorcluster, "Position"=w440:T2, "Top"=w442:i32, "Left"=w434:i32)
                    n220 = Add(x=w442, y=w441) -> (x+y=w439:i32)
                    n221 = Add(x=w434, y=w432) -> (x+y=w433:i32)
                    n222 = Bundle By Name(cluster=w440, "Top"=w439, "Left"=w433) -> (w438:T2)
                    n223 = invoke class="GObj" method="Move"(reference=w443, error in=w436, "position"=w438) -> (error out=w435:errorcluster)  [unwired: 3 in, 5 out]
                  }
                  n224 = Merge Errors(w427) -> (w422:errorcluster)
                }
              }
            }
            frame "Choice 2" {
              # "OUTSIDE"
              n225 = case shown="\"Right\"" w451 {
                tunnel: [w452 w493 w523 w547] -> w445
                tunnel: w448 -> [w456 w492 w521 w544]
                tunnel: w449 -> [w457 w490 w519 w545]
                tunnel: w447 -> [w455 w484 w522 w543]
                tunnel: w450 -> [w454 w491 w520 w546]
                tunnel: w446 -> [w453 w487 _ w542]
                frame "Left", Default {
                  n226 = property class="GrowFunc"(reference=w455) -> ("MasterRect"=w463:T3)  [unwired: 1 in, 2 out]
                  n227 = property class="Term"(reference=w454) -> ("MasterRect"=w462:T3)  [unwired: 1 in, 2 out]
                  n228 = Unbundle By Name(w463) -> ("Right"=w460:i16)
                  n229 = Unbundle By Name(w462) -> ("Left"=w461:i16)
                  n230 = Subtract(x=w461, y=w460) -> (x-y=w464:i16)
                  n231 = Add(x=w464, y=w453) -> (x+y=w459:i32)
                  n232 = for {
                    tunnel: w459 -> [w472]
                    tunnel: [w467] -> w458 mode=indexing
                    tunnel: w457 -> [w466] mode=indexing
                    tunnel: w456 -> [w465]
                    n233 = property class="GObj"(reference=w466, error in=w465) -> (reference out=w474:refnum<vi>, error out=w468:errorcluster, "Position"=w471:T2, "Left"=w473:i32)
                    n234 = Add(x=w473, y=w472) -> (x+y=w470:i32)
                    n235 = Bundle By Name(cluster=w471, "Left"=w470) -> (w469:T2)
                    n236 = invoke class="GObj" method="Move"(reference=w474, error in=w468, "position"=w469) -> (error out=w467:errorcluster)  [unwired: 3 in, 5 out]
                  }
                  n237 = Merge Errors(w458) -> (w452:errorcluster)
                }
                frame "Top" {
                  n238 = property class="GrowFunc"(reference=w484) -> ("Terms[]"=w483:refnum<vi>[])  [unwired: 1 in, 2 out]
                  n239 = property class="GrowFunc"(reference=w484) -> ("MasterRect"=w486:T3)  [unwired: 1 in, 2 out]
                  n240 = property class="Term"(reference=w491) -> ("MasterRect"=w480:T3)  [unwired: 1 in, 2 out]
                  n241 = Index Array(array=w483) -> (element=w478:refnum<vi>)  [unwired: 1 in]
                  n242 = Unbundle By Name(w486) -> ("Bottom"=w485:i16)
                  n243 = property class="Term"(reference=w478) -> ("MasterRect"=w475:T3)  [unwired: 1 in, 2 out]
                  n244 = call <vilib>:"RectCentroid.vi"("rect"=w480) -> ("point"=w481:cluster{"x":i16, "y":i16})
                  n245 = Unbundle By Name(w480) -> ("Top"=w494:i16)
                  n246 = Unbundle By Name(w481) -> ("x"=w479:i16)
                  n247 = call <vilib>:"RectCentroid.vi"("rect"=w475) -> ("point"=w477:cluster{"x":i16, "y":i16})
                  n248 = Subtract(x=w494, y=w485) -> (x-y=w495:i16)
                  n249 = Unbundle By Name(w477) -> ("x"=w476:i16)
                  n250 = Add(x=w495, y=w487) -> (x+y=w488:i32)
                  n251 = Subtract(x=w479, y=w476) -> (x-y=w482:i16)
                  n252 = for {
                    tunnel: w492 -> [w502]
                    tunnel: w490 -> [w501] mode=indexing
                    tunnel: [w500] -> w489 mode=indexing
                    tunnel: w488 -> [w499]
                    tunnel: w482 -> [w496]
                    n253 = property class="GObj"(reference=w501, error in=w502) -> (reference out=w508:refnum<vi>, error out=w503:errorcluster, "Position"=w506:T2, "Top"=w507:i32, "Left"=w498:i32)
                    n254 = Add(x=w507, y=w499) -> (x+y=w505:i32)
                    n255 = Add(x=w498, y=w496) -> (x+y=w497:i32)
                    n256 = Bundle By Name(cluster=w506, "Top"=w505, "Left"=w497) -> (w504:T2)
                    n257 = invoke class="GObj" method="Move"(reference=w508, error in=w503, "position"=w504) -> (error out=w500:errorcluster)  [unwired: 3 in, 5 out]
                  }
                  n258 = Merge Errors(w489) -> (w493:errorcluster)
                }
                frame "Bottom" {
                  n259 = property class="GrowFunc"(reference=w522) -> ("Terms[]"=w517:refnum<vi>[])  [unwired: 1 in, 2 out]
                  n260 = property class="Term"(reference=w520) -> ("MasterRect"=w511:T3)  [unwired: 1 in, 2 out]
                  n261 = Index Array(array=w517) -> (element=w516:refnum<vi>)  [unwired: 1 in]
                  n262 = property class="Term"(reference=w516) -> ("MasterRect"=w515:T3)  [unwired: 1 in, 2 out]
                  n263 = call <vilib>:"RectCentroid.vi"("rect"=w511) -> ("point"=w512:cluster{"x":i16, "y":i16})
                  n264 = Unbundle By Name(w512) -> ("x"=w510:i16)
                  n265 = call <vilib>:"RectCentroid.vi"("rect"=w515) -> ("point"=w514:cluster{"x":i16, "y":i16})
                  n266 = Unbundle By Name(w514) -> ("x"=w513:i16)
                  n267 = Subtract(x=w510, y=w513) -> (x-y=w509:i16)
                  n268 = for {
                    tunnel: w521 -> [w527]
                    tunnel: w519 -> [w526] mode=indexing
                    tunnel: [w525] -> w518 mode=indexing
                    tunnel: w509 -> [w524]
                    n269 = property class="GObj"(reference=w526, error in=w527) -> (reference out=w533:refnum<vi>, error out=w528:errorcluster, "Position"=w531:T2, "Left"=w532:i32)
                    n270 = Add(x=w532, y=w524) -> (x+y=w530:i32)
                    n271 = Bundle By Name(cluster=w531, "Left"=w530) -> (w529:T2)
                    n272 = invoke class="GObj" method="Move"(reference=w533, error in=w528, "position"=w529) -> (error out=w525:errorcluster)  [unwired: 3 in, 5 out]
                  }
                  n273 = Merge Errors(w518) -> (w523:errorcluster)
                }
                frame "Right" {
                  n274 = property class="GrowFunc"(reference=w543) -> ("MasterRect"=w540:T3)  [unwired: 1 in, 2 out]
                  n275 = property class="Term"(reference=w546) -> ("MasterRect"=w539:T3)  [unwired: 1 in, 2 out]
                  n276 = Absolute Value(x=w542) -> (abs(x)=w535:i32)
                  n277 = Unbundle By Name(w539) -> ("Right"=w538:i16)
                  n278 = Unbundle By Name(w540) -> ("Left"=w537:i16)
                  n279 = Subtract(x=w538, y=w537) -> (x-y=w541:i16)
                  n280 = Add(x=w541, y=w535) -> (x+y=w534:i32)
                  n281 = for {
                    tunnel: w545 -> [w557] mode=indexing
                    tunnel: w534 -> [w554]
                    tunnel: w544 -> [w550]
                    tunnel: [w548] -> w536 mode=indexing
                    n282 = property class="GObj"(reference=w557, error in=w550) -> (reference out=w556:refnum<vi>, error out=w549:errorcluster, "Position"=w553:T2, "Left"=w555:i32)
                    n283 = Add(x=w555, y=w554) -> (x+y=w552:i32)
                    n284 = Bundle By Name(cluster=w553, "Left"=w552) -> (w551:T2)
                    n285 = invoke class="GObj" method="Move"(reference=w556, error in=w549, "position"=w551) -> (error out=w548:errorcluster)  [unwired: 3 in, 5 out]
                  }
                  n286 = Merge Errors(w536) -> (w547:errorcluster)
                }
              }
            }
          }
        }
      }
    }
  }
  "error out" <- w9
